vi "receive.vi"(0 "ISubnet in":refnum<class "ISubnet.lvclass">, 11 "error in (no error)":errorcluster) -> (4 "ISubnet out":refnum<class "ISubnet.lvclass">, 6 "ValidCRC":i32, 8 "InvalidCRC":i32, 10 "Messages":i32, 14 "CRCIssues":T1[](array[typedef]) {"Data" format="%02x"}, 15 "error out":errorcluster)   [LabVIEW 2016, in "ISubnet.lvclass"]
uses:
  ISubnet.lvclass
  Common_RT_Modbus/DataTypes/RxFrame.ctl
  Common_RT_Modbus/RTModbus.lvlib
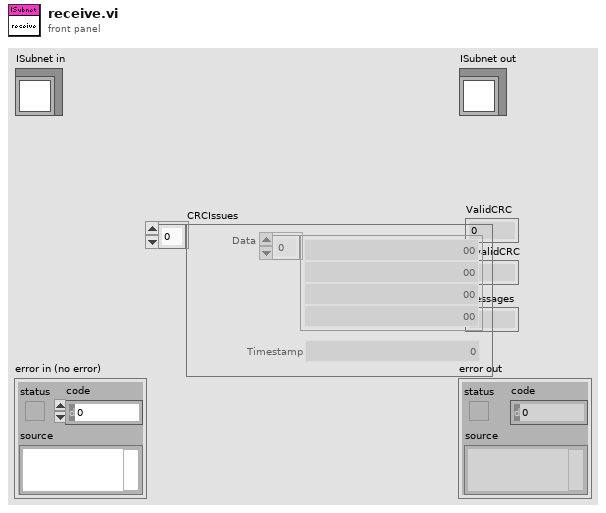
[diagram p1: front panel]
types:
  T1 = typedef "RTModbus.lvlib/RxFrame.ctl" = cluster{"Data":u8[], "Timestamp":u64}
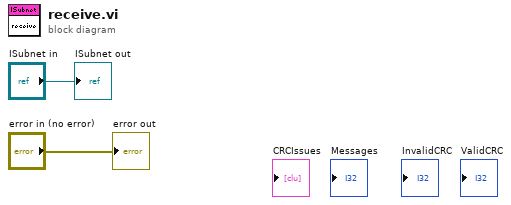
[diagram p0: block diagram]
diagram:
  "error out" <- "error in (no error)"
  "ISubnet out" <- "ISubnet in"
